vi "RobotToRunMode.vi"() -> (3 "Mode Out":T1)   [LabVIEW 2017]
uses:
  RunMode.ctl
  <vilib>/Rock Robotics/WPI/DriverStation/WPI_DriverStationRobotMode2.ctl
  RobotSubsystem.lvclass
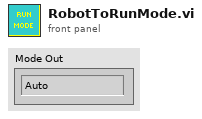
[diagram p1: front panel]
types:
  T1 = typedef "RobotSubsystem.lvclass/RunMode.ctl" = enum16{"Auto", "Teleop", "Disabled"}
  T2 = typedef "WPI_DriverStationRobotMode2.ctl" = enum16{"Autonomous Disabled", "Autonomous Enabled", "Teleop Disabled", "Teleop Enabled", "Disconnected", "Finish", "Test Disabled", "Test Enabled", "Emergency Stopped"}
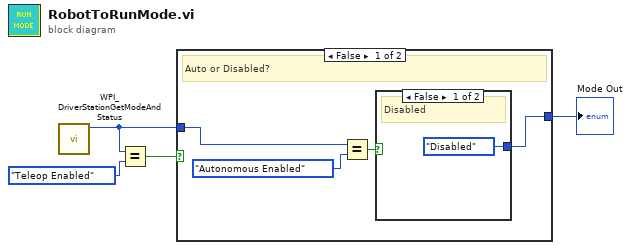
[diagram p0: block diagram]
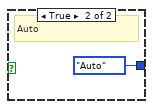
[diagram p2: hidden frame]
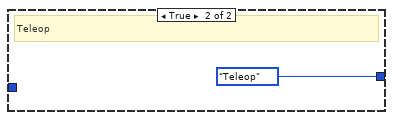
[diagram p3: hidden frame]
diagram:
  n1 = call <vilib>:"WPI_DriverStationGetModeAndStatus.vi"() -> ("Robot Mode"=w2:T2)  [unwired: 10 in, 1 out]
  n2 = Equal?(x=w2, y=WPI_DriverStationRobotMode2."Teleop Enabled" ("Robot Mode")) -> (x = y?=w4:bool)
  n3 = case shown="False" w4 {
    tunnel: [w8 RunMode."Teleop" ("Mode")] -> w1
    tunnel: w2 -> [w5 _]
    frame False {
      # "Auto or Disabled?"
      n4 = Equal?(x=w5, y=WPI_DriverStationRobotMode2."Autonomous Enabled" ("Robot Mode")) -> (x = y?=w7:bool)
      n5 = case shown="False" w7 {
        tunnel: [RunMode."Disabled" ("Mode") RunMode."Auto" ("Mode")] -> w8
        frame False {
          # "Disabled"
        }
        frame True {
          # "Auto"
        }
      }
    }
    frame True {
      # "Teleop"
    }
  }
  "Mode Out" <- w1
